vi "ExtractFolder.vi"(1 "path":path) -> (0 "Array":string[](array[string]))   [LabVIEW 2018]
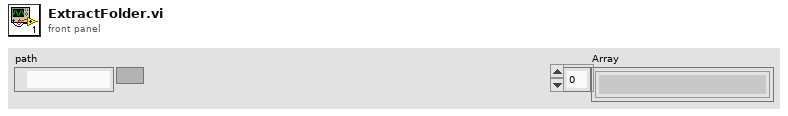
[diagram p1: front panel]
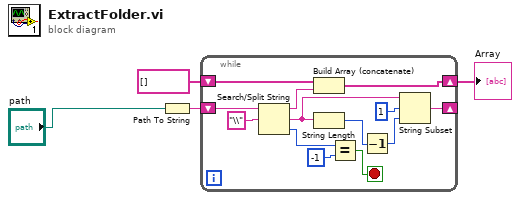
[diagram p0: block diagram]
diagram:
  n1 = Path To String(path="path") -> (string=w4:string)
  n2 = while {
    shift-right: [w9] -> _
    shift-left: w4 -> [w17]
    shift-right: [w15] -> w2
    shift-left: string[] [] -> [w14]
    stop <- w13 stop-if-true
    n3 = Search/Split String(string=w17, search string/char (-)="\\") -> (substring before match=w16:string, match + rest of string=w7:string, offset of match=w12:i32)  [unwired: 1 in]
    n4 = Build Array (concatenate)(w14, w16) -> (w15:string[])
    n5 = String Length(string=w7) -> (length=w6:i32)
    n6 = Equal?(x=w12, y=-1) -> (x = y?=w13:bool)
    n7 = Decrement(x=w6) -> (x-1=w5:i32)
    n8 = String Subset(string=w7, offset (0)=1, length (rest)=w5) -> (substring=w9:string)
  }
  "Array" <- w2
